vi "Autonomous Independent.vi"   [LabVIEW 2017]
doc: "This VI is called when autonomous begins, and will automatically be terminated when autonomous ends. You can carry out timed or sensor driven robot movement independently without needing to return to the caller."
uses:
  <vilib>/Rock Robotics/WPI/Utilities/WPI_GetSetVariantRefNum.vi
  <vilib>/Rock Robotics/Network Tables/NT Read String.vi
  Robot Global Data.vi
  <vilib>/Rock Robotics/Network Tables/NT Write Numeric Array.vi
panel:
  # "Be sure to right-click and choose Data Operations>>Make Current Value default if you want to save the array values with the VI"
types:
  T1 = typedef "WPI_JoystickDevRef.ctl" = cluster{"Device":T2}
  T2 = typedef "WPI_JoystickDeviceEnum.ctl" = enum16{"USB 0", "USB 1", "USB 2", "USB 3", "USB 4", "USB 5"}
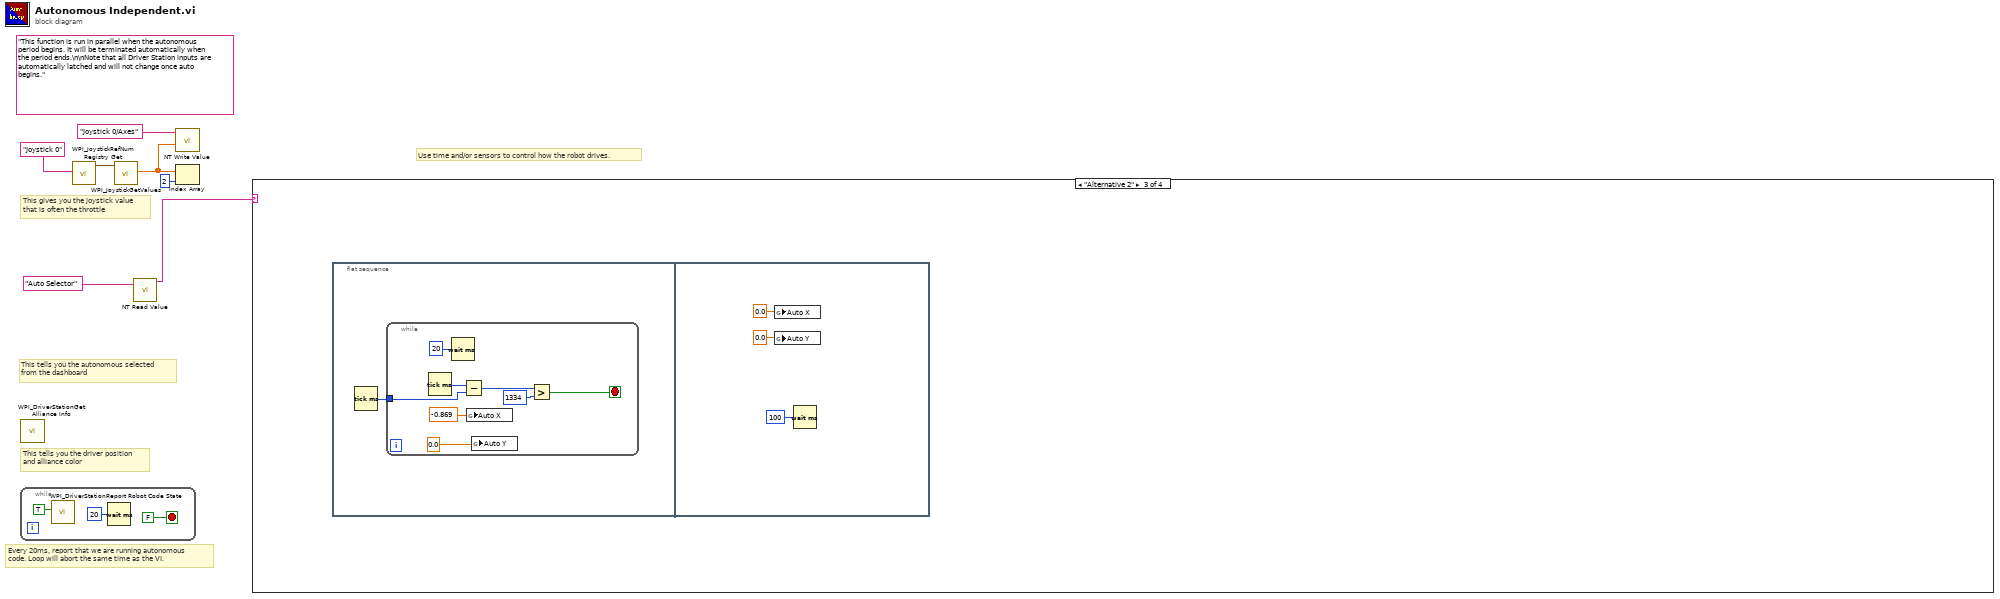
[diagram p0: block diagram]
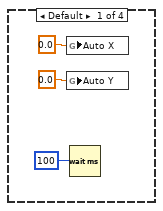
[diagram p2: hidden frame]
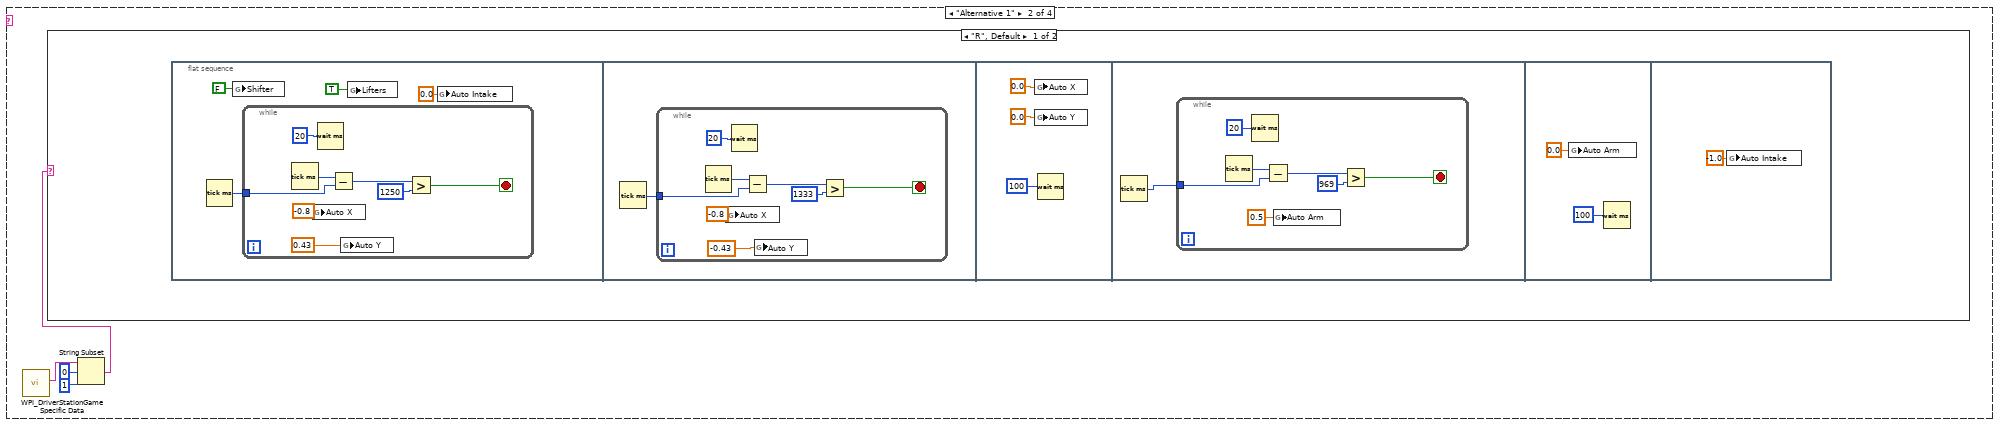
[diagram p3: hidden frame]
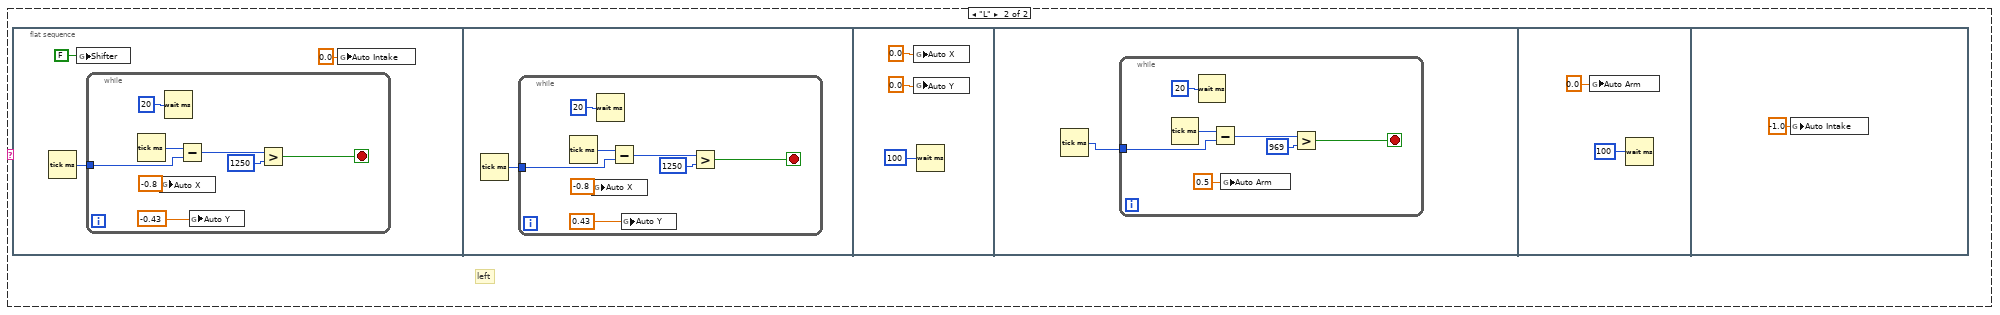
[diagram p4: hidden frame]
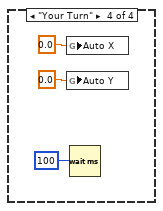
[diagram p5: hidden frame]
diagram:
  (unwired) "This function is run in parallel when the autonomous period begins. It will be terminated automatically when the period ends.\n\nNote that all Driver Station inputs are automatically latched and will not change once auto begins."
  # "This tells you the autonomous selected\nfrom the dashboard"
  # "Every 20ms, report that we are running autonomous\ncode. Loop will abort the same time as the VI."
  # "This gives you the joystick value\nthat is often the throttle"
  # "Use time and/or sensors to control how the robot drives."
  # "This tells you the driver position\nand alliance color"
  n1 = while {
    stop <- FALSE stop-if-true
    n2 = call <vilib>:"WPI_DriverStationReport Robot Code State.vi"("Autonomous"=TRUE) -> ()  [unwired: 10 in, 1 out]
    n3 = Wait (ms)(milliseconds to wait=u32 20) -> ()  [unwired: 1 out]
  }
  n4 = call <vilib>:"WPI_DriverStationGet Alliance Info.vi"() -> ()  [unwired: 12 out]
  n5 = call <vilib>:"WPI_JoystickRefNum Registry Get.vi"("refnum name"="Joystick 0") -> ("JoystickDevRef"=w6:T1)  [unwired: 1 in, 9 out]
  n6 = call <vilib>:"WPI_JoystickGetValues.vi"("JoystickDevRef"=w6) -> ("Axes"=w2:dbl[])  [unwired: 6 in, 4 out]
  n7 = call-poly <vilib>:"NT Read Value.vi"("Name"="Auto Selector") -> ("String"=w3:string)  [unwired: 9 in, 1 out]
  n8 = call-poly <vilib>:"NT Write Value.vi"("Numeric Array"=w2, "Name"="Joystick 0/Axes") -> ()  [unwired: 9 in, 1 out]
  n9 = Index Array(array=w2, index=2) -> ()  [unwired: 1 out]
  n10 = case shown="\"Alternative 2\"" w3 {
    frame Default {
      n11 = global write "Robot Global Data.vi" "Auto X"(0.0) -> ()
      n12 = global write "Robot Global Data.vi" "Auto Y"(0.0) -> ()
      n13 = Wait (ms)(milliseconds to wait=u32 100) -> ()  [unwired: 1 out]
    }
    frame "Alternative 1" {
      n14 = call <vilib>:"WPI_DriverStationGame Specific Data.vi"() -> ("Game Specific Data"=w17:string)  [unwired: 11 in]
      n15 = String Subset(string=w17, offset (0)=0, length (rest)=1 ("length (rest)")) -> (substring=w14:string)
      n16 = case shown="\"R\", Default" w14 {
        frame "R", Default {
          n17 = flat-sequence {
            frame #0 {
              n18 = Tick Count (ms)() -> (millisecond timer value=w21:u32)
              n19 = global write "Robot Global Data.vi" "Shifter"(FALSE ("Shifter")) -> ()
              n20 = while {
                tunnel: w21 -> [w29]
                stop <- w25 stop-if-true
                n21 = Tick Count (ms)() -> (millisecond timer value=w28:u32)
                n22 = global write "Robot Global Data.vi" "Auto X"(-0.8) -> ()
                n23 = Wait (ms)(milliseconds to wait=u32 20) -> ()  [unwired: 1 out]
                n24 = Subtract(x=w28, y=w29) -> (x-y=w27:u32)
                n25 = global write "Robot Global Data.vi" "Auto Y"(0.43) -> ()
                n26 = Greater?(x=w27, y=u32 1250) -> (0:w25:bool)
              }
              n27 = global write "Robot Global Data.vi" "Lifters"(TRUE ("Shifter")) -> ()
              n28 = global write "Robot Global Data.vi" "Auto Intake"(0.0 ("Auto Arm")) -> ()
            }
            frame #1 {
              n29 = Tick Count (ms)() -> (millisecond timer value=w30:u32)
              n30 = while {
                tunnel: w30 -> [w38]
                stop <- w34 stop-if-true
                n31 = Tick Count (ms)() -> (millisecond timer value=w37:u32)
                n32 = global write "Robot Global Data.vi" "Auto X"(-0.8) -> ()
                n33 = Wait (ms)(milliseconds to wait=u32 20) -> ()  [unwired: 1 out]
                n34 = Subtract(x=w37, y=w38) -> (x-y=w36:u32)
                n35 = global write "Robot Global Data.vi" "Auto Y"(-0.43) -> ()
                n36 = Greater?(x=w36, y=u32 1333) -> (0:w34:bool)
              }
            }
            frame #2 {
              n37 = global write "Robot Global Data.vi" "Auto X"(0.0) -> ()
              n38 = global write "Robot Global Data.vi" "Auto Y"(0.0) -> ()
              n39 = Wait (ms)(milliseconds to wait=u32 100) -> ()  [unwired: 1 out]
            }
            frame #3 {
              n40 = Tick Count (ms)() -> (millisecond timer value=w42:u32)
              n41 = while {
                tunnel: w42 -> [w49]
                stop <- w45 stop-if-true
                n42 = Tick Count (ms)() -> (millisecond timer value=w48:u32)
                n43 = Wait (ms)(milliseconds to wait=u32 20) -> ()  [unwired: 1 out]
                n44 = Subtract(x=w48, y=w49) -> (x-y=w47:u32)
                n45 = global write "Robot Global Data.vi" "Auto Arm"(0.5 ("Auto Arm")) -> ()
                n46 = Greater?(x=w47, y=u32 969) -> (0:w45:bool)
              }
            }
            frame #4 {
              n47 = global write "Robot Global Data.vi" "Auto Arm"(0.0 ("Auto Arm")) -> ()
              n48 = Wait (ms)(milliseconds to wait=u32 100) -> ()  [unwired: 1 out]
            }
            frame #5 {
              n49 = global write "Robot Global Data.vi" "Auto Intake"(-1.0 ("Auto Arm")) -> ()
            }
          }
        }
        frame "L" {
          # "left"
          n50 = flat-sequence {
            frame #0 {
              n51 = Tick Count (ms)() -> (millisecond timer value=w55:u32)
              n52 = global write "Robot Global Data.vi" "Shifter"(FALSE ("Shifter")) -> ()
              n53 = while {
                tunnel: w55 -> [w63]
                stop <- w59 stop-if-true
                n54 = Tick Count (ms)() -> (millisecond timer value=w62:u32)
                n55 = global write "Robot Global Data.vi" "Auto X"(-0.8) -> ()
                n56 = Wait (ms)(milliseconds to wait=u32 20) -> ()  [unwired: 1 out]
                n57 = Subtract(x=w62, y=w63) -> (x-y=w61:u32)
                n58 = global write "Robot Global Data.vi" "Auto Y"(-0.43) -> ()
                n59 = Greater?(x=w61, y=u32 1250) -> (0:w59:bool)
              }
              n60 = global write "Robot Global Data.vi" "Auto Intake"(0.0 ("Auto Arm")) -> ()
            }
            frame #1 {
              n61 = Tick Count (ms)() -> (millisecond timer value=w64:u32)
              n62 = while {
                tunnel: w64 -> [w72]
                stop <- w68 stop-if-true
                n63 = Tick Count (ms)() -> (millisecond timer value=w71:u32)
                n64 = global write "Robot Global Data.vi" "Auto X"(-0.8) -> ()
                n65 = Wait (ms)(milliseconds to wait=u32 20) -> ()  [unwired: 1 out]
                n66 = Subtract(x=w71, y=w72) -> (x-y=w70:u32)
                n67 = global write "Robot Global Data.vi" "Auto Y"(0.43) -> ()
                n68 = Greater?(x=w70, y=u32 1250) -> (0:w68:bool)
              }
            }
            frame #2 {
              n69 = global write "Robot Global Data.vi" "Auto X"(0.0) -> ()
              n70 = global write "Robot Global Data.vi" "Auto Y"(0.0) -> ()
              n71 = Wait (ms)(milliseconds to wait=u32 100) -> ()  [unwired: 1 out]
            }
            frame #3 {
              n72 = Tick Count (ms)() -> (millisecond timer value=w76:u32)
              n73 = while {
                tunnel: w76 -> [w83]
                stop <- w79 stop-if-true
                n74 = Tick Count (ms)() -> (millisecond timer value=w82:u32)
                n75 = Wait (ms)(milliseconds to wait=u32 20) -> ()  [unwired: 1 out]
                n76 = Subtract(x=w82, y=w83) -> (x-y=w81:u32)
                n77 = global write "Robot Global Data.vi" "Auto Arm"(0.5 ("Auto Arm")) -> ()
                n78 = Greater?(x=w81, y=u32 969) -> (0:w79:bool)
              }
            }
            frame #4 {
              n79 = global write "Robot Global Data.vi" "Auto Arm"(0.0 ("Auto Arm")) -> ()
              n80 = Wait (ms)(milliseconds to wait=u32 100) -> ()  [unwired: 1 out]
            }
            frame #5 {
              n81 = global write "Robot Global Data.vi" "Auto Intake"(-1.0 ("Auto Arm")) -> ()
            }
          }
        }
      }
    }
    frame "Alternative 2" {
      n82 = flat-sequence {
        frame #0 {
          n83 = Tick Count (ms)() -> (millisecond timer value=w87:u32)
          n84 = while {
            tunnel: w87 -> [w95]
            stop <- w91 stop-if-true
            n85 = Tick Count (ms)() -> (millisecond timer value=w94:u32)
            n86 = Wait (ms)(milliseconds to wait=u32 20) -> ()  [unwired: 1 out]
            n87 = Subtract(x=w94, y=w95) -> (x-y=w93:u32)
            n88 = global write "Robot Global Data.vi" "Auto X"(-0.869) -> ()
            n89 = global write "Robot Global Data.vi" "Auto Y"(0.0) -> ()
            n90 = Greater?(x=w93, y=u32 1334) -> (0:w91:bool)
          }
        }
        frame #1 {
          n91 = global write "Robot Global Data.vi" "Auto X"(0.0) -> ()
          n92 = global write "Robot Global Data.vi" "Auto Y"(0.0) -> ()
          n93 = Wait (ms)(milliseconds to wait=u32 100) -> ()  [unwired: 1 out]
        }
      }
    }
    frame "Your Turn" {
      n94 = global write "Robot Global Data.vi" "Auto X"(0.0) -> ()
      n95 = global write "Robot Global Data.vi" "Auto Y"(0.0) -> ()
      n96 = Wait (ms)(milliseconds to wait=u32 100) -> ()  [unwired: 1 out]
    }
  }
